vi "carrier_waveforms.vi"(5 "Modulation info":T7={"Fs full"=0.0, "Fs high"=0.0, "Fs low"=0.0, "Read size"=0, "FFT size low"=5000, "df low"=5000.0, "High carriers"=[], "Low carriers"=[], "Hi channels at low"=[7]} {"Hi channels at low" min=0 step=1; "Low carriers" format="%#_6p"; "High carriers" format="%#_6p"}, 7 "ilemt_config":T1={"IO params"={"Conversion"={"Rate"=4.0, "In channels"=2, "Out channels"=4}, "Carriers"={"Phase shift"=180.0, "Levels"=[[0.8, 0.8, 0.8], [0.03, 0.03, 0.03]], "Delay samples"=73.15}}, "High rate STFT"={"Win param"=101.5, "Window type"=61, "Win order"=2, "DFT size"=64, "Channels"=[7], "Oversample"=64}, "Low rate STFT"={"Win param"=120.0, "Window type"=61, "Win order"=8, "DFT size"=64, "Channels"=[7], "Oversample"=64}, "Filtering"={"Hum"={"Frequency"=0.0, "Tc"=0.0, "Limit"=101.5, "FFT filter"=FALSE, "Detrend mode"=enum."Robust linear", "Enable"=FALSE}, "Kalman"={"Process noise"=101.5, "Measure noise"=101.5, "Unlock m noise"=101.5, "Mode"=enum."FFT"}, "Distortion"={"LF cut"=101.5, "Tc"=3.0, "Limit"=101.5, "FFT filter"=FALSE, "Detrend mode"=enum."Robust linear", "Enable"=FALSE}, "Lowpass"={"Frequency"=0.0, "Order"=0, "Enable"=FALSE}, "Impulse"={"Win order"=102, "Locked limit"=101.5, "Locked count"=102, "Threshold Tc"=101.5, "Thresh sigmas"=101.5, "Thresh min"=101.5, "After"=0, "Detrend"=FALSE, "Enable"=FALSE}}} {"Filtering"."Impulse"."Thresh min" format="%#_3p"; "Filtering"."Impulse"."Threshold Tc" format="%#_3p"; "Filtering"."Impulse"."Locked limit" format="%#_3p"; "Filtering"."Impulse"."Thresh sigmas" format="%#_3p"; "Filtering"."Lowpass"."Frequency" format="%#_4p"; "Filtering"."Distortion"."Limit" format="%#_3p"; "Filtering"."Distortion"."LF cut" format="%#_3p"; "Filtering"."Kalman"."Unlock m noise" format="%#_3p"; "Filtering"."Kalman"."Measure noise" format="%#_3p"; "Filtering"."Kalman"."Process noise" format="%#_3p"; "Filtering"."Hum"."Limit" format="%#_3p"; "Filtering"."Hum"."Frequency" format="%#_4p"; "Low rate STFT"."Oversample" min=1 step=1; "Low rate STFT"."Channels" min=0 step=1; "Low rate STFT"."DFT size" min=1 step=1; "Low rate STFT"."Window type" items=["Rectangle"=0, "Hanning"=1, "Hamming"=2, "Blackman-Harris"=3, "Exact Blackman"=4, "Blackman"=5, "Flat Top"=6, "4 Term B-Harris "=7, "7 Term B-Harris"=8, "Low Sidelobe"=9, "Blackman Nuttall"=11, "Triangle"=30, "Bartlett-Hanning"=31, "Bohman"=32, "Parzen"=33, "Welch"=34, "Kaiser"=60, "Dolph-Chebyshev"=61, "Gaussian"=62]; "High rate STFT"."Oversample" min=1 step=1; "High rate STFT"."Channels" min=0 step=1; "High rate STFT"."DFT size" min=1 step=1; "High rate STFT"."Window type" items=["Rectangle"=0, "Hanning"=1, "Hamming"=2, "Blackman-Harris"=3, "Exact Blackman"=4, "Blackman"=5, "Flat Top"=6, "4 Term B-Harris "=7, "7 Term B-Harris"=8, "Low Sidelobe"=9, "Blackman Nuttall"=11, "Triangle"=30, "Bartlett-Hanning"=31, "Bohman"=32, "Parzen"=33, "Welch"=34, "Kaiser"=60, "Dolph-Chebyshev"=61, "Gaussian"=62]; "IO params"."Carriers"."Levels" min=0.0 step=0.1; "IO params"."Conversion"."Rate" format="%#_8g"}) -> (2 "Output data":i32[][](array[numeric]), 3 "Source waveforms":waveform(dbl)[](graph))   [LabVIEW 2014]
uses:
  modulation_info.ctl
  ilemt_config.ctl
  IO_params.ctl
  stft_params.ctl
  <vilib>/Analysis/4window.llb/windowTd.ctl
  filter_params.ctl
  detrend_mode.ctl
  <vilib>/Analysis/2dsp.llb/Inverse Real FFT.vi
  <vilib>/measure/NI_MABase.lvlib
  <vilib>/Analysis/NI_AALPro.lvlib
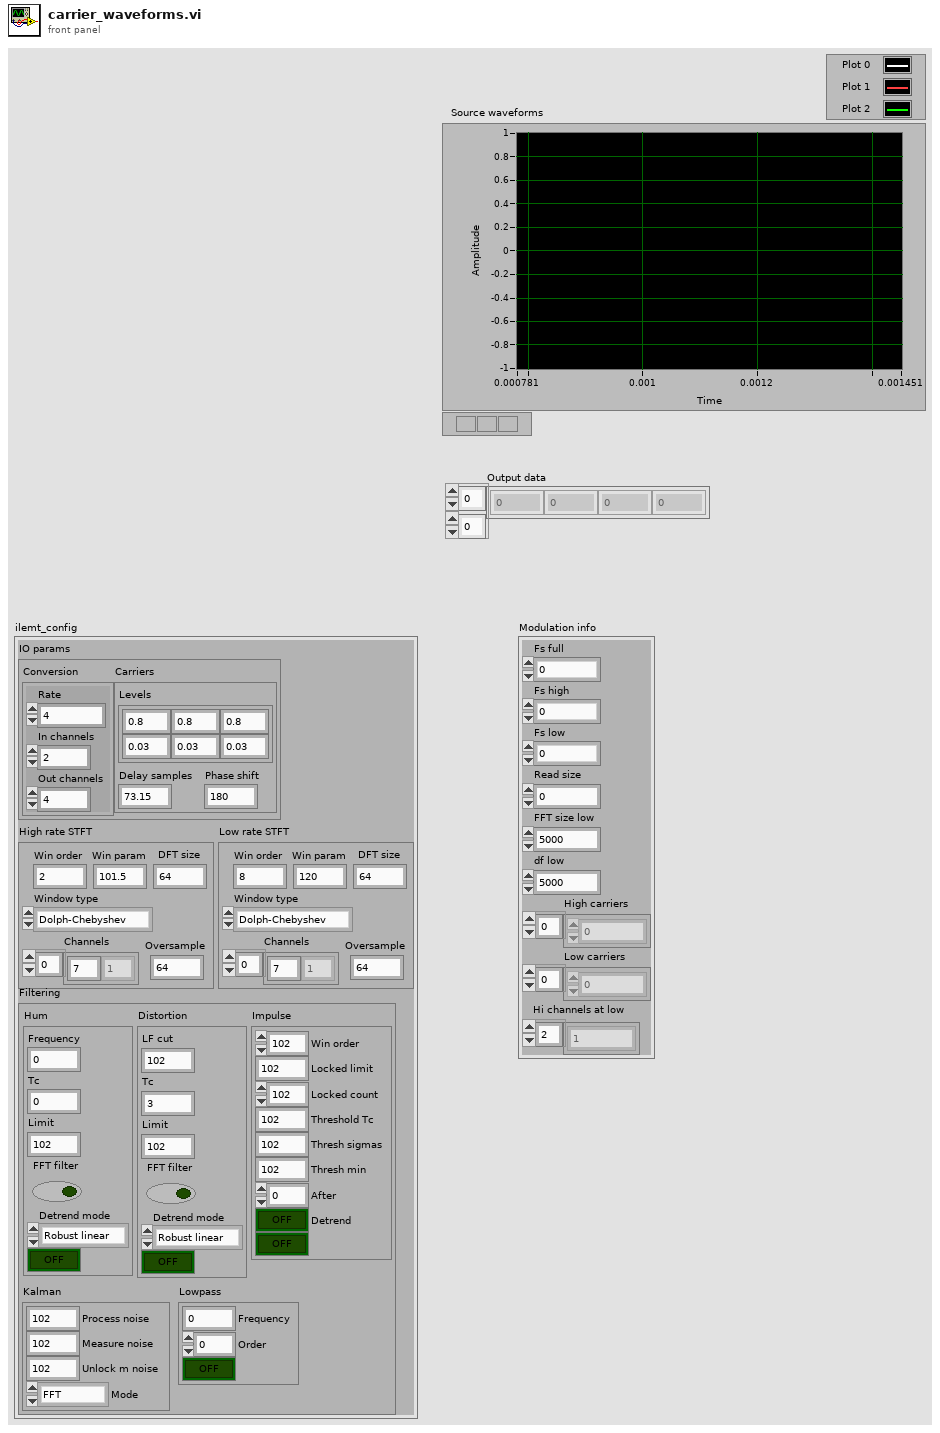
[diagram p1: front panel]
types:
  T1 = typedef "ilemt_config.ctl" = cluster{"IO params":T2, "High rate STFT":T3, "Low rate STFT":T3, "Filtering":T5}
  T2 = typedef "IO_params.ctl" = cluster{"Conversion":cluster{"Rate":dbl, "In channels":u32, "Out channels":u32}, "Carriers":cluster{"Phase shift":dbl, "Levels":dbl[][], "Delay samples":dbl}}
  T3 = typedef "stft_params.ctl" = cluster{"Win param":dbl, "Window type":T4, "Win order":i32, "DFT size":i32, "Channels":i32[], "Oversample":i32}
  T4 = typedef "NI_AALPro.lvlib/windowTd.ctl" = u32
  T5 = typedef "filter_params.ctl" = cluster{"Hum":cluster{"Frequency":dbl, "Tc":dbl, "Limit":dbl, "FFT filter":bool, "Detrend mode":T6, "Enable":bool}, "Kalman":cluster{"Process noise":dbl, "Measure noise":dbl, "Unlock m noise":dbl, "Mode":enum16{"FFT", "KF demod"}}, "Distortion":cluster{"LF cut":dbl, "Tc":dbl, "Limit":dbl, "FFT filter":bool, "Detrend mode":T6, "Enable":bool}, "Lowpass":cluster{"Frequency":dbl, "Order":i32, "Enable":bool}, "Impulse":cluster{"Win order":i32, "Locked limit":dbl, "Locked count":i32, "Threshold Tc":dbl, "Thresh sigmas":dbl, "Thresh min":dbl, "After":i32, "Detrend":bool, "Enable":bool}}
  T6 = typedef "detrend_mode.ctl" = enum16{"Zero mean", "Linear", "Robust linear"}
  T7 = typedef "modulation_info.ctl" = cluster{"Fs full":dbl, "Fs high":dbl, "Fs low":dbl, "Read size":i32, "FFT size low":i32, "df low":dbl, "High carriers":dbl[], "Low carriers":dbl[], "Hi channels at low":i32[]}
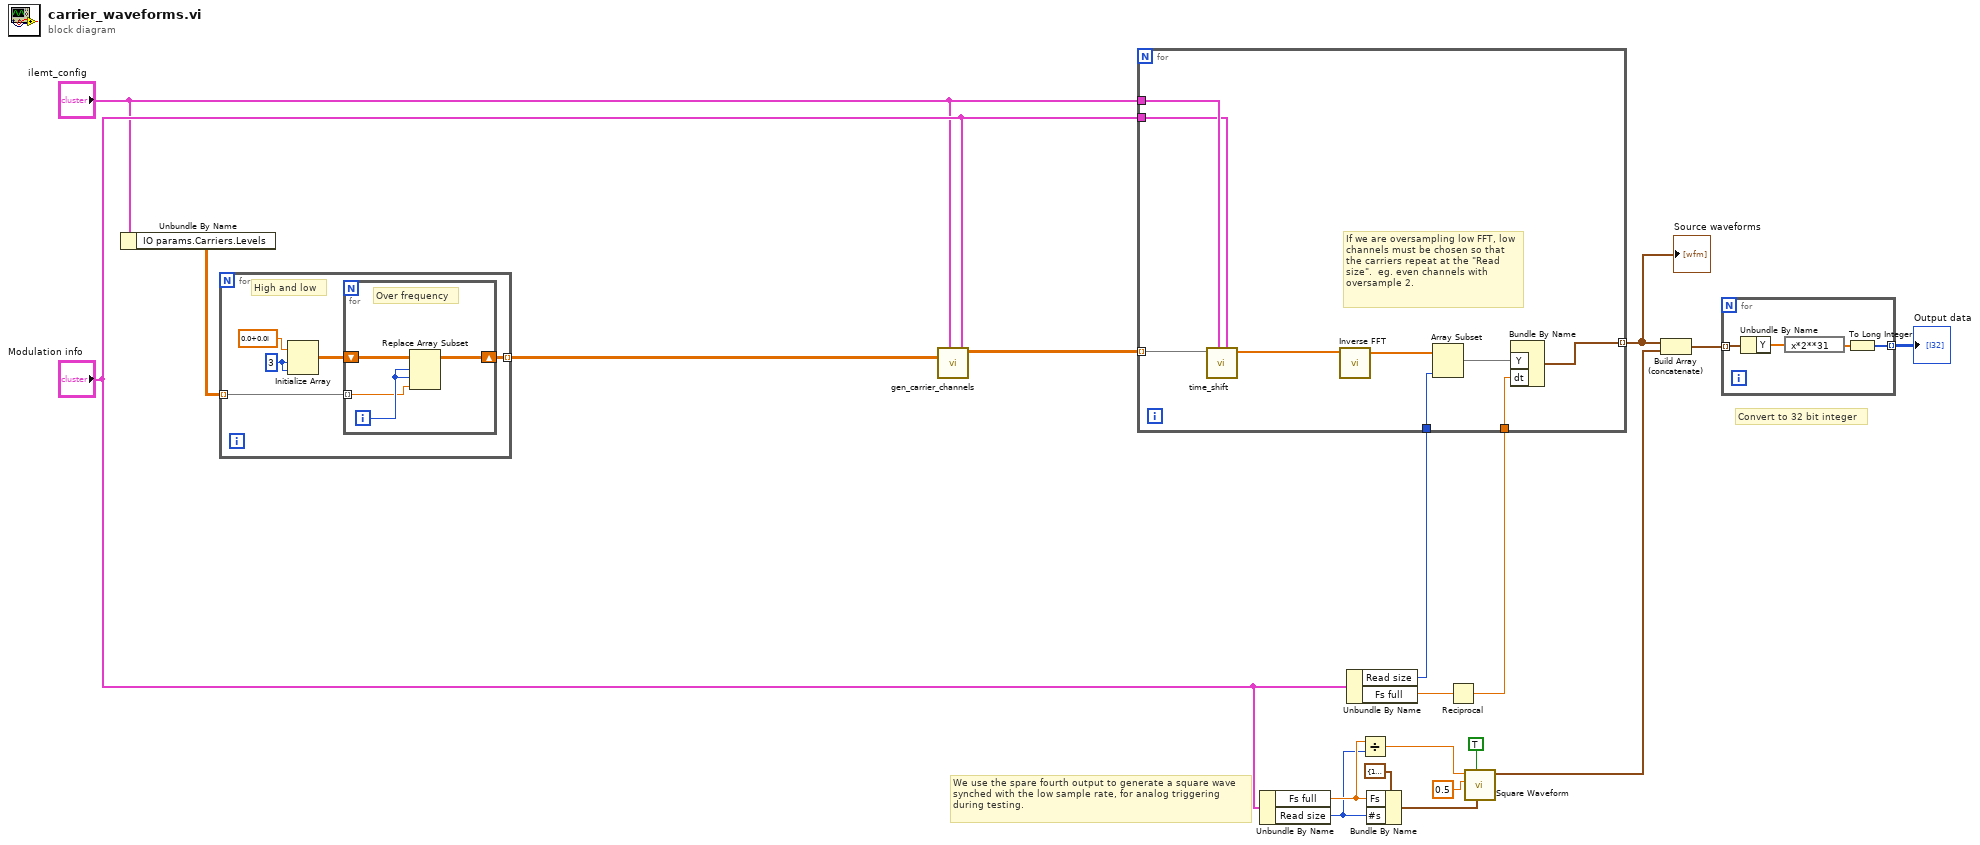
[diagram p0: block diagram]
diagram:
  # "Convert to 32 bit integer"
  # "We use the spare fourth output to generate a square wave synched with the low sample rate, for analog triggering during testing."
  n1 = Unbundle By Name("ilemt_config") -> ("IO params.Carriers.Levels"=w2:dbl[][])
  n2 = for {
    tunnel: w2 -> [w21] mode=indexing
    tunnel: [w20] -> w1 mode=indexing
    w24 = 3 ("dimension size")
    # "High and low"
    n3 = Initialize Array(cdb 0.0+0.0i, w24, w24) -> (w22:cdb[][])
    n4 = for {
      tunnel: w21 -> [w26] mode=indexing
      shift-right: [w25] -> w20
      shift-left: w22 -> [w28]
      i -> [w27]
      # "Over frequency"
      n5 = Replace Array Subset(array=w28, new element=w26, index (row)=w27, index (col)=w27) -> (w25:cdb[][])
    }
  }
  n6 = call "gen_carrier_channels.vi"("Modulation info"="Modulation info", "ilemt_config"="ilemt_config", "Source amplitudes"=w1) -> ("Carrier DFT"=w5:cdb[][])  [unwired: 8 in]
  n7 = Unbundle By Name("Modulation info") -> ("Fs full"=w18:dbl, "Read size"=w6:i32)
  n8 = Unbundle By Name("Modulation info") -> ("Read size"=w9:i32, "Fs full"=w8:dbl)
  n9 = Divide(x=w18, y=w6) -> (x/y=w15:dbl)
  n10 = Bundle By Name(cluster=cluster{"Fs":dbl, "#s":dbl} {"Fs"=1000.0, "#s"=1000.0} ("sampling info"), "Fs"=w18, "#s"=w6) -> (w16:cluster{"Fs":dbl, "#s":dbl})
  n11 = Reciprocal(x=w8) -> (1/x=w7:dbl)
  n12 = for {
    tunnel: [w37] -> w12 mode=indexing
    tunnel: w9 -> [w33]
    tunnel: w7 -> [w32]
    tunnel: "ilemt_config" -> [w31]
    tunnel: "Modulation info" -> [w30]
    tunnel: w5 -> [w29] mode=indexing
    # "If we are oversampling low FFT, low channels must be chosen so that the carriers repeat at the \"Read size\".  eg. even channels with oversample 2."
    n13 = call "time_shift.vi"("Modulation info"=w30, "ilemt_config"=w31, "Array in"=w29) -> ("Array out"=w34:cdb[])  [unwired: 8 in]
    n14 = call-poly <vilib>:"Inverse FFT.vi"("FFT {X}"=w34) -> ("X"=w36:dbl[])  [unwired: 9 in, 1 out]
    n15 = Array Subset(array=w36, length=w33) -> (w35:dbl[])  [unwired: 1 in]
    n16 = Bundle By Name("Y"=w35, "dt"=w32) -> (w37:waveform(dbl))  [unwired: 1 in]
  }
  "Source waveforms" <- w12
  n17 = call <vilib>:"Square Waveform.vi"("sampling info"=w16, "reset signal"=TRUE, "amplitude"=0.5, "frequency"=w15) -> ("signal out"=w13:waveform(dbl))  [unwired: 6 in, 1 out]
  n18 = Build Array (concatenate)(w12, w13) -> (w11:waveform(dbl)[])
  n19 = for {
    tunnel: w11 -> [w41] mode=indexing
    tunnel: [w38] -> w10 mode=indexing
    n20 = Unbundle By Name(w41) -> ("Y"=w40:dbl[])
    n21 = expression code="x*2**31"(w40) -> (w39:dbl[])
    n22 = To Long Integer(number=w39) -> (32bit integer=w38:i32[])
  }
  "Output data" <- w10
